vi "EXO1_DataRead&Plot_backup.vi"() -> ()   [LabVIEW 2012]
uses:
  <vilib>/addons/database/Connection.llb/DB Tools Open Connec (Path).vi
  <vilib>/addons/database/NI_Database_API.lvlib
panel:
  out "Plot 4":cluster{dbl[], dbl[]}[](graph)
  out "Plot 3":cluster{dbl[], dbl[]}[](graph)
  out "Plot 2":cluster{dbl[], dbl[]}[](graph)
  out "Plot":cluster{dbl[], dbl[]}[](graph)
  in  "Start time":timestamp
  in  "End time":timestamp
  out "Data List":string[][](table)
  out "error out":errorcluster
  in  "Table chosen":string="EXO"
  in  "stop":bool
  # "EXO Data Read & Plots"
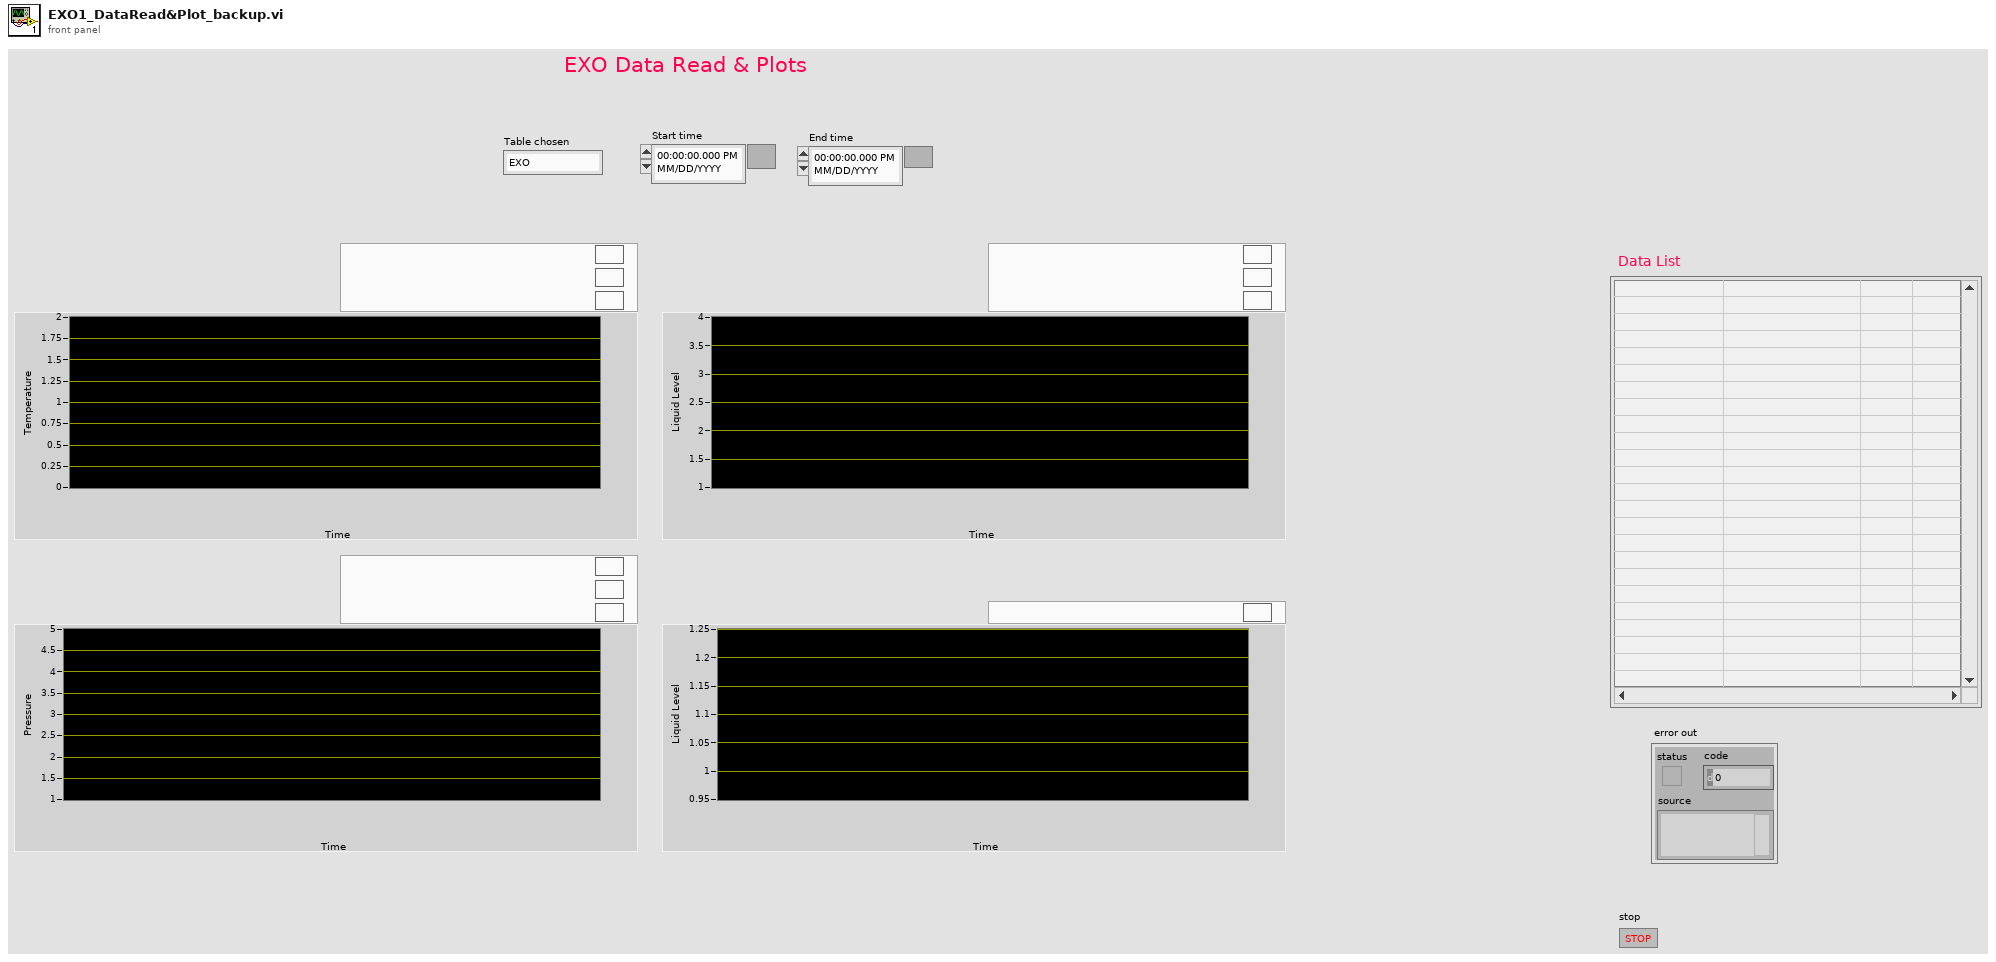
[diagram p1: front panel]
types:
  T1 = typedef "NI_Database_API.lvlib/Conn ObjectReference.ctl" = refnum<k1>
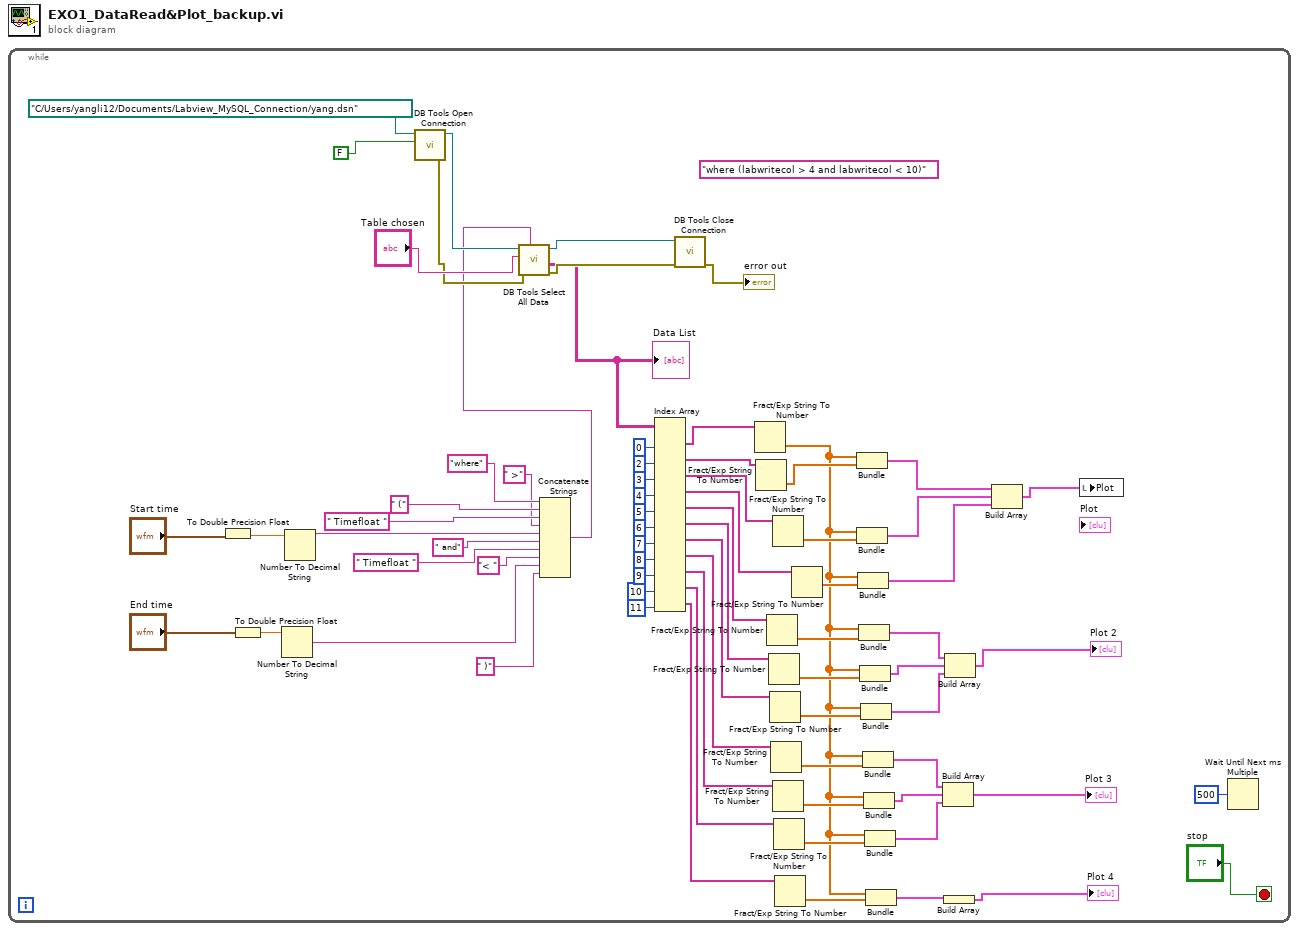
[diagram p0: block diagram]
diagram:
  n1 = while {
    stop <- "stop" stop-if-true
    (unwired) "where (labwritecol > 4 and labwritecol < 10)" ("condition")
    n2 = To Double Precision Float(number="Start time") -> (double precision float=w52:dbl)
    n3 = To Double Precision Float(number="End time") -> (double precision float=w47:dbl)
    n4 = Number To Decimal String(number=w47) -> (decimal integer string=w46:string)  [unwired: 1 out]
    n5 = Number To Decimal String(number=w52) -> (decimal integer string=w51:string)  [unwired: 1 out]
    n6 = call-poly <vilib>:"DB Tools Open Connection.vi"("prompt? (F)"=FALSE, "connection information"=path "C:/Users/yangli12/Documents/Labview_MySQL_Connection/yang.dsn") -> ("error out"=w66:errorcluster, "connection reference"=w68:T1)  [unwired: 6 in]
    n7 = Concatenate Strings("where", " (", " Timefloat " ("string"), " >" ("string"), w51, " and", " Timefloat ", "< " ("string"), w46, " )") -> (w44:string)
    n8 = call <vilib>:"DB Tools Select All Data.vi"("optional clause"=w44, "error in (no error)"=w66, "table"="Table chosen", "connection reference"=w68) -> ("error out"=w65:errorcluster, "data"=w63:string[][], "connection reference out"=w64:T1)  [unwired: 1 in, 1 out]
    "Data List" <- w63
    n9 = Index Array(array=w63, index (col) #1=0 ("disabled index (col)"), index (col) #2=2 ("index (col)"), index (col) #3=3 ("index (col)"), index (col) #4=4 ("index (col)"), index (col) #5=5 ("index (col)"), index (col) #6=6 ("index (col)"), index (col) #7=7 ("index (col)"), index (col) #8=8 ("index (col)"), index (col) #9=9 ("index (col)"), index (col) #10=10 ("index (col)"), index (col) #11=11 ("index (col)")) -> (element #1=w60:string[], element #2=w40:string[], element #3=w43:string[], element #4=w28:string[], element #5=w25:string[], element #6=w24:string[], element #7=w23:string[], element #8=w15:string[], element #9=w14:string[], element #10=w13:string[], element #11=w5:string[])  [unwired: 11 in]
    n10 = call <vilib>:"DB Tools Close Connection.vi"("error in (no error)"=w65, "connection reference"=w64) -> ("error out"=→"error out":errorcluster)  [unwired: 5 in]
    n11 = Fract/Exp String To Number(string=w60) -> (number=w3:dbl[])  [unwired: 4 out]
    n12 = Fract/Exp String To Number(string=w40) -> (number=w59:dbl[])  [unwired: 4 out]
    n13 = Fract/Exp String To Number(string=w25) -> (number=w22:dbl[])  [unwired: 4 out]
    n14 = Fract/Exp String To Number(string=w24) -> (number=w21:dbl[])  [unwired: 4 out]
    n15 = Fract/Exp String To Number(string=w23) -> (number=w20:dbl[])  [unwired: 4 out]
    n16 = Fract/Exp String To Number(string=w15) -> (number=w12:dbl[])  [unwired: 4 out]
    n17 = Fract/Exp String To Number(string=w43) -> (number=w42:dbl[])  [unwired: 4 out]
    n18 = Fract/Exp String To Number(string=w14) -> (number=w11:dbl[])  [unwired: 4 out]
    n19 = Fract/Exp String To Number(string=w13) -> (number=w10:dbl[])  [unwired: 4 out]
    n20 = Fract/Exp String To Number(string=w5) -> (number=w4:dbl[])  [unwired: 4 out]
    n21 = Fract/Exp String To Number(string=w28) -> (number=w27:dbl[])  [unwired: 4 out]
    n22 = Bundle "Bundle"(w3, w59) -> (w39:cluster{dbl[], dbl[]})  [unwired: 1 in]
    n23 = Bundle "Bundle"(w3, w42) -> (w38:cluster{dbl[], dbl[]})  [unwired: 1 in]
    n24 = Bundle "Bundle"(w3, w27) -> (w26:cluster{dbl[], dbl[]})  [unwired: 1 in]
    n25 = Bundle "Bundle"(w3, w22) -> (w19:cluster{dbl[], dbl[]})  [unwired: 1 in]
    n26 = Bundle "Bundle"(w3, w21) -> (w18:cluster{dbl[], dbl[]})  [unwired: 1 in]
    n27 = Bundle "Bundle"(w3, w20) -> (w17:cluster{dbl[], dbl[]})  [unwired: 1 in]
    n28 = Bundle "Bundle"(w3, w12) -> (w9:cluster{dbl[], dbl[]})  [unwired: 1 in]
    n29 = Bundle "Bundle"(w3, w11) -> (w8:cluster{dbl[], dbl[]})  [unwired: 1 in]
    n30 = Bundle "Bundle"(w3, w10) -> (w7:cluster{dbl[], dbl[]})  [unwired: 1 in]
    n31 = Bundle "Bundle"(w3, w4) -> (w2:cluster{dbl[], dbl[]})  [unwired: 1 in]
    n32 = Build Array(w9, w8, w7) -> (→"Plot 3":cluster{dbl[], dbl[]}[])
    n33 = Build Array(w2) -> (→"Plot 4":cluster{dbl[], dbl[]}[])
    n34 = Build Array(w19, w18, w17) -> (→"Plot 2":cluster{dbl[], dbl[]}[])
    n35 = Build Array(w39, w38, w26) -> (w37:cluster{dbl[], dbl[]}[])
    n36 = local write "Plot"(w37) -> ()
    n37 = Wait Until Next ms Multiple(millisecond multiple=u32 500) -> ()  [unwired: 1 out]
  }
